vi "Delta Mode Measurements.vi"() -> ()   [LabVIEW 2023]
doc: "Demonstrates the fundamentals of the Queued Message Handler design pattern in LabVIEW. A queued message handler, in its simplest form, is composed of two loops. The Event Handling Loop responds to user interface events by enqueuing \"messages\" on a message queue. These messages are dequeued in the Message Handling Loop. Note that the Message Handling Loop is also capable of sending messages to itself."
uses:
  <instrlib>/Keithley 622x LV 2009/Configure/2182 -A/Low Level/Typedefs/KE2182 -- Voltage Ranges.ctl
  <instrlib>/Keithley 622x LV 2009/Configure/2182 -A/Low Level/Typedefs/KE2182 -- Filter Type.ctl
  <instrlib>/Keithley 622x LV 2009/Configure/2182 -A/Low Level/Typedefs/KE2182 -- Filter Count.ctl
  <instrlib>/Keithley 622x LV 2009/Configure/2182 -A/Low Level/Typedefs/KE2182 -- Filter Window.ctl
  <instrlib>/Keithley 622x LV 2009/Configure/2182 -A/Low Level/Typedefs/KE2182 -- NPLCs.ctl
  <instrlib>/Keithley 622x LV 2009/Configure/Delta PDelta DCon Modes/Typedefs/KE622x -- Delta Mode Params.ctl
  <instrlib>/Keithley 622x LV 2009/Configure/Delta PDelta DCon Modes/Low Level/Typedefs/KE622x -- Delta PDelta Mode High Level.ctl
  <instrlib>/Keithley 622x LV 2009/Configure/Delta PDelta DCon Modes/Low Level/Typedefs/KE622x -- Delta PDelta Mode Low Level.ctl
  <instrlib>/Keithley 622x LV 2009/Configure/Delta PDelta DCon Modes/Low Level/Typedefs/KE622x -- Delta DCon Mode Delay.ctl
  <instrlib>/Keithley 622x LV 2009/Configure/Delta PDelta DCon Modes/Low Level/Typedefs/KE622x -- Delta PDelta Mode Num Cycles Mode.ctl
  <instrlib>/Keithley 622x LV 2009/Configure/Delta PDelta DCon Modes/Low Level/Typedefs/KE622x -- Delta PDelta Mode Num Cycles.ctl
  <instrlib>/Keithley 622x LV 2009/Configure/Units/Typedefs/KE622x -- Voltage Meas Units.ctl
  Program Files/National Instruments/LabVIEW 2023/examples/Design Patterns/Queued Message Handler/support/QMH Fundamentals - Message Cluster.ctl
  <vilib>/Utility/error.llb/Error Cluster From Error Code.vi
  Lakeshore 336/Global temperature.vi
  <vilib>/ErrorRing/Error Ring.xnode
  <instrlib>/Keithley 622x LV 2009/Keithley 622x.lvlib
panel:
  out "Number of points":i32
  out "Array - Numeric":dbl[][](array[numeric]) format="%#_11g"
  out "XY Graph":cluster{dbl[], dbl[]}(graph)
  out "Temperature":dbl format="%.4f"
  in  "Voltage Meas Units":T1
  in  "Stop Delta Mode":bool
  out "Amplitude":dbl
  in  "Exit":bool
  in  "Start Acquisition":bool
  in  "Delta Mode Params In":T2={"High Level (A)"=0.001, "Low Level (A)"=-0.001, "Delay (s)"=0.002, "Num Cycles Mode"=enum."Infinite", "Finite Count"=10, "Abort On\nCompliance?"=FALSE, "Cold Swithing\nMode Enabled?"=FALSE} {"Finite Count" min=2 max=65536; "Low Level (A)" min=-0.105 max=0.0 format="%.3p"; "High Level (A)" min=0.0 max=0.105 format="%.3p"; "Delay (s)" min=0.001 max=9999.999 format="%.3f"}
  in  "2812 -A Params In":T13={"Auto Range?"=FALSE, "Man / Selected\nRange"=enum."10mV", "Enable Digital\nFilter?"=FALSE, "Filter Type"=enum."Moving", "Filter Count"=10, "Filter\nWindow (%)"=0.01, "Enable Analog\nFilter?"=FALSE, "NPLCs"=2} {"Filter\nWindow (%)" min=0.0 max=10.0 step=0.01 format="%.2f"; "Filter Count" min=1 max=100; "NPLCs" min=1 max=10}
  in  "Start Delta Mode":bool
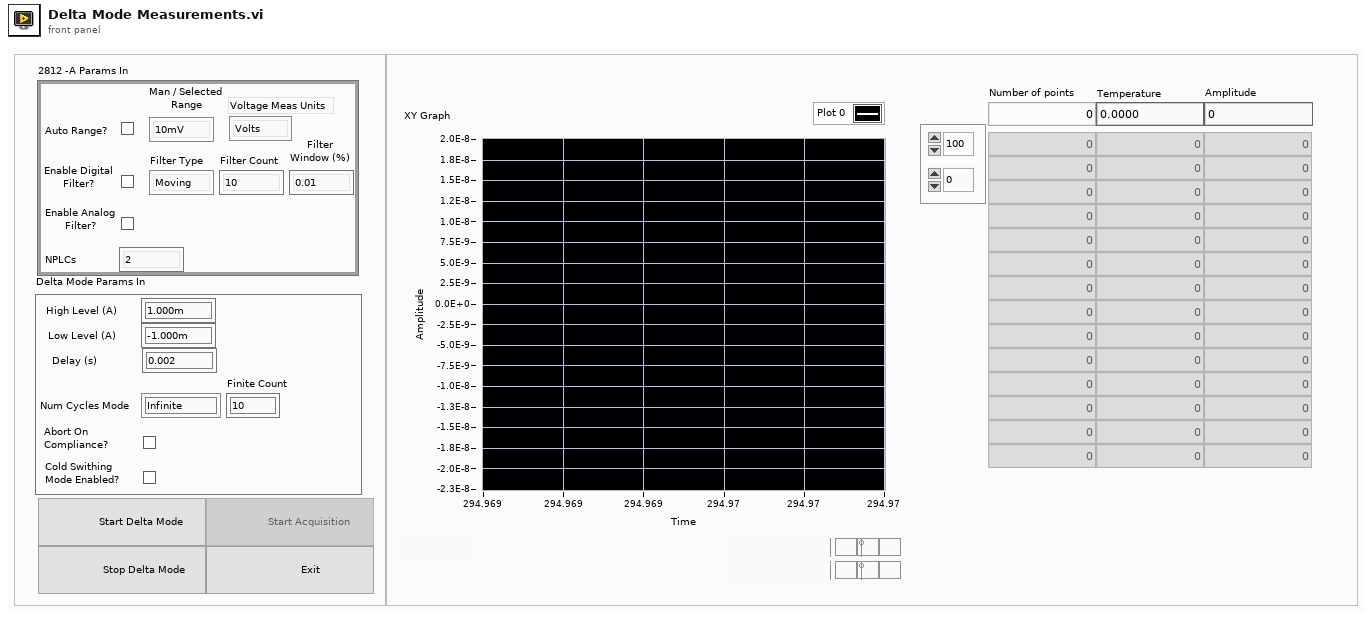
[diagram p1: front panel]
types:
  T1 = typedef "Keithley 622x.lvlib/KE622x -- Voltage Meas Units.ctl" = enum16{"Volts", "Ohms", "Watts", "Siemens"}
  T2 = typedef "Keithley 622x.lvlib/KE622x -- Delta Mode Params.ctl" = cluster{"High Level (A)":T3, "Low Level (A)":T4, "Delay (s)":T5, "Num Cycles Mode":T6, "Finite Count":T7, "Abort On\nCompliance?":bool, "Cold Swithing\nMode Enabled?":bool}
  T3 = typedef "Keithley 622x.lvlib/KE622x -- Delta PDelta Mode High Level.ctl" = dbl
  T4 = typedef "Keithley 622x.lvlib/KE622x -- Delta PDelta Mode Low Level.ctl" = dbl
  T5 = typedef "Keithley 622x.lvlib/KE622x -- Delta DCon Mode Delay.ctl" = dbl
  T6 = typedef "Keithley 622x.lvlib/KE622x -- Delta PDelta Mode Num Cycles Mode.ctl" = enum16{"Finite Count", "Infinite"}
  T7 = typedef "Keithley 622x.lvlib/KE622x -- Delta PDelta Mode Num Cycles.ctl" = u32
  T8 = typedef "Keithley 622x.lvlib/KE2182 -- Voltage Ranges.ctl" = enum16{"10mV", "100mV", "1V", "10V", "100V"}
  T9 = typedef "Keithley 622x.lvlib/KE2182 -- Filter Type.ctl" = enum16{"Moving", "Repeat"}
  T10 = typedef "Keithley 622x.lvlib/KE2182 -- Filter Count.ctl" = u32
  T11 = typedef "Keithley 622x.lvlib/KE2182 -- Filter Window.ctl" = dbl
  T12 = typedef "Keithley 622x.lvlib/KE2182 -- NPLCs.ctl" = u32
  T13 = cluster{"Auto Range?":bool, "Man / Selected\nRange":T8, "Enable Digital\nFilter?":bool, "Filter Type":T9, "Filter Count":T10, "Filter\nWindow (%)":T11, "Enable Analog\nFilter?":bool, "NPLCs":T12}
  T14 = enum8{"Enabled", "Disabled", "Disabled and Grayed Out"}
  T15 = typedef "QMH Fundamentals - Message Cluster.ctl" = cluster{"Message":string, "Message Data":variant}
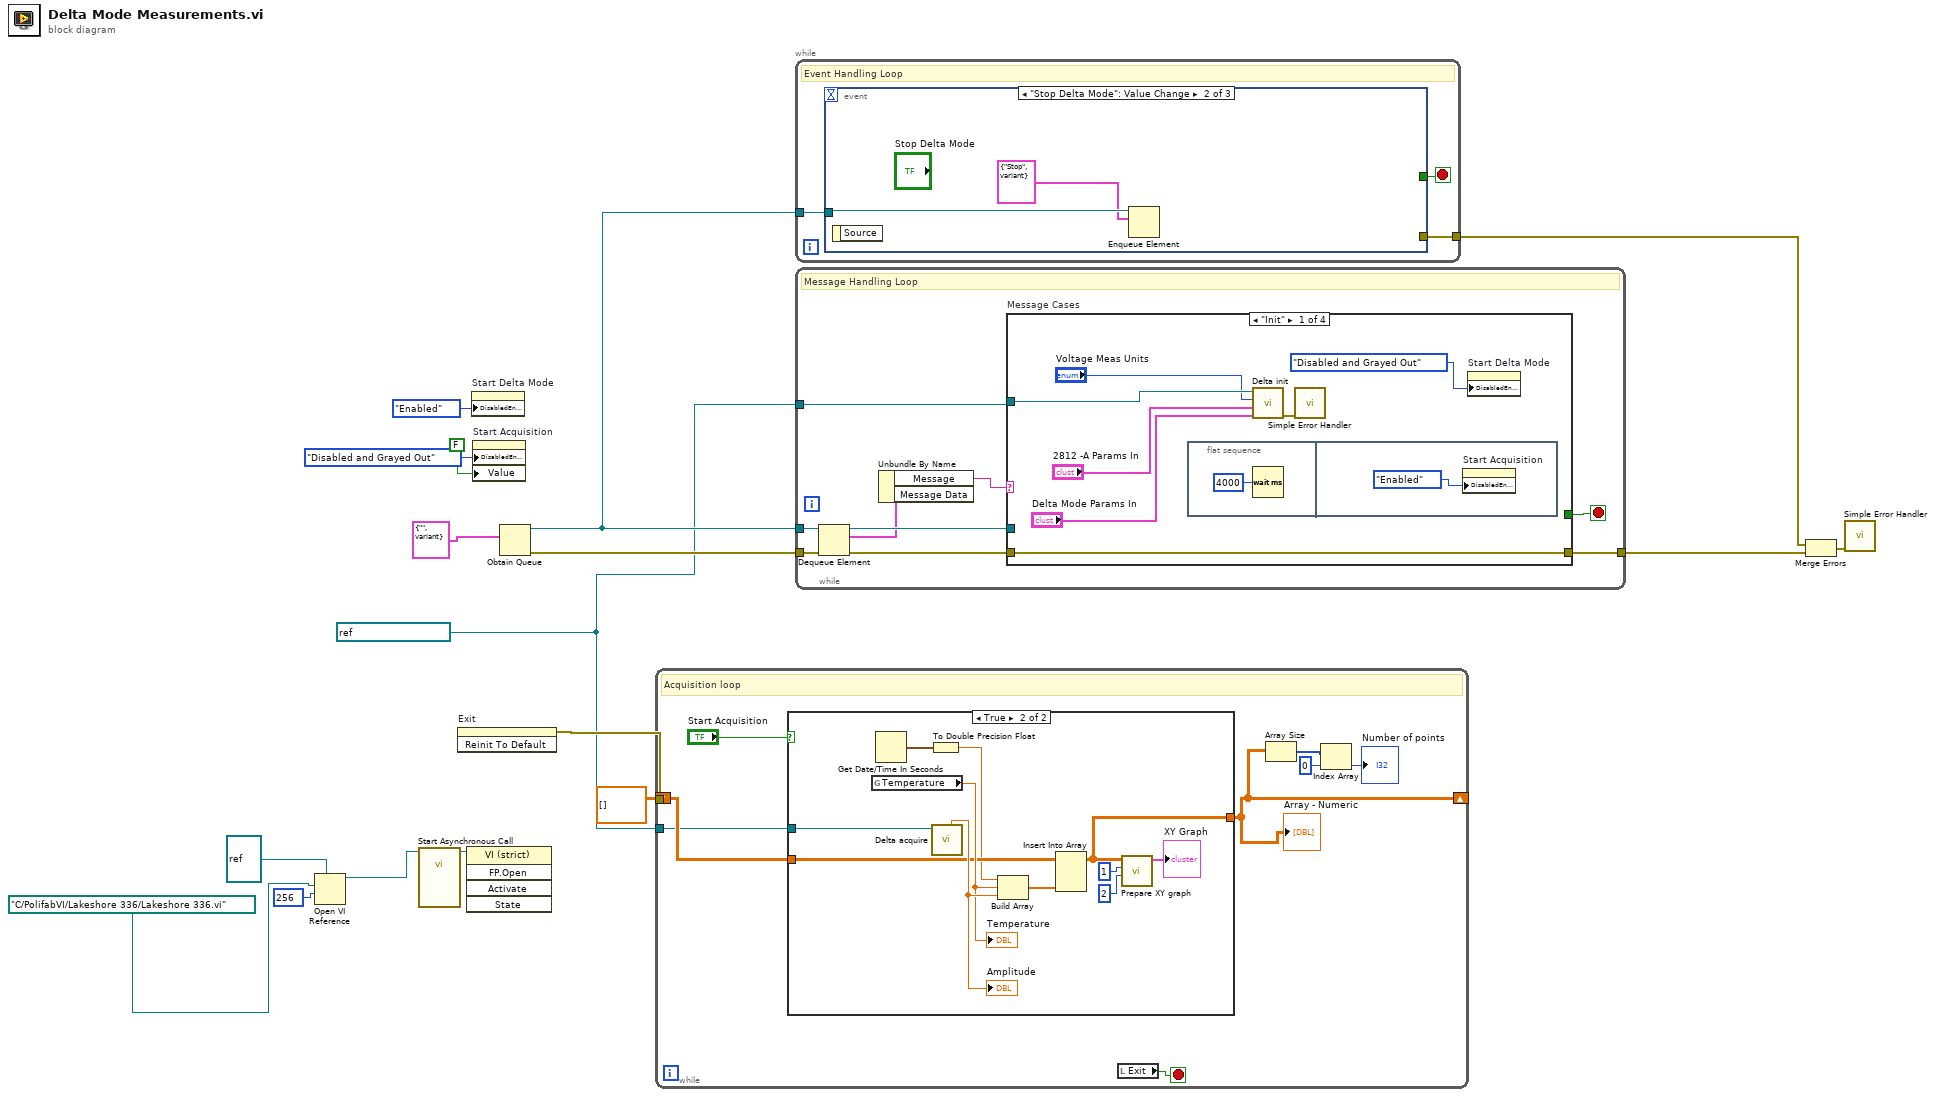
[diagram p0: block diagram]
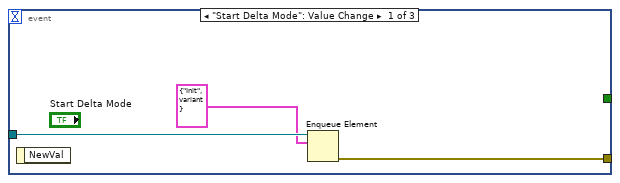
[diagram p3: hidden frame]
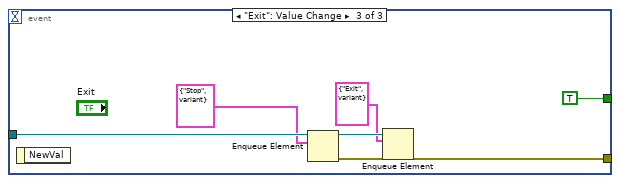
[diagram p4: hidden frame]
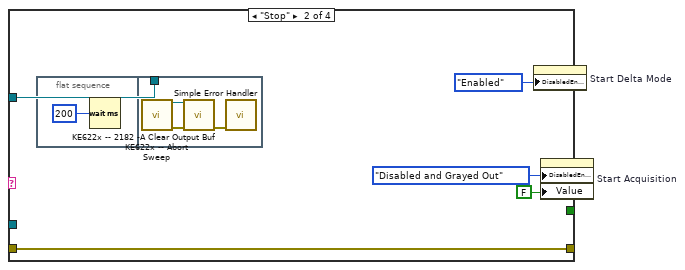
[diagram p5: hidden frame]
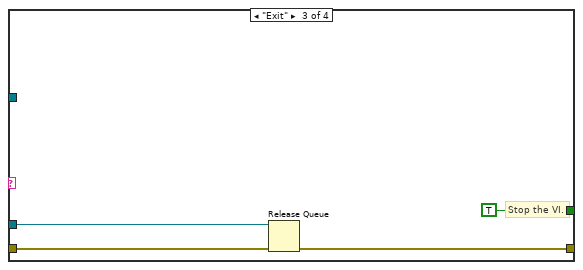
[diagram p6: hidden frame]
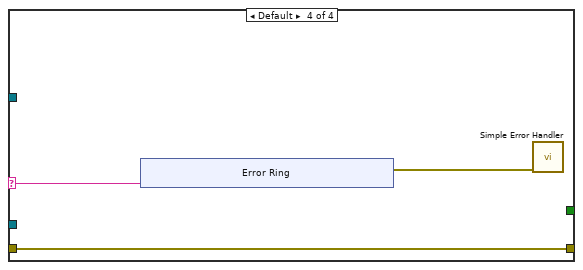
[diagram p7: hidden frame]
diagram:
  w1 = refnum<visa-resource-name> "GPIB0::12::INSTR" ("622x Resource")
  n1 = Open VI Reference(type specifier VI Refnum (for type only)=refnum<vi> refnum, vi path=path "C:/PolifabVI/Lakeshore 336/Lakeshore 336.vi", options=256) -> (vi reference=w4:refnum<vi>)  [unwired: 3 in, 1 out]
  n2 = call-by-ref "Start Asynchronous Call"(reference=w4) -> (reference out=w3:refnum<vi>)  [unwired: 2 in, 2 out]
  n3 = invoke on="Exit" class="Bool (strict)" method="Reinit To Default"() -> (error out=w11:errorcluster)  [unwired: 3 in, 2 out]
  n4 = invoke class="VI (strict)" method="FP.Open"(reference=w3) -> ()  [unwired: 4 in, 5 out]
  n5 = property on="Start Delta Mode" class="Bool"("DisabledEnum"=T14."Enabled" ("Disabled")) -> ()  [unwired: 2 in, 2 out]
  n6 = property on="Start Acquisition" class="Bool (strict)"("DisabledEnum"=T14."Disabled and Grayed Out" ("Disabled"), "Value"=FALSE ("Start Acquisition")) -> ()  [unwired: 2 in, 2 out]
  n7 = Obtain Queue(element data type=T15 {"Message"="", "Message Data"=variant} ("Message Cluster")) -> (queue out=w12:refnum<queue>, error out=w13:errorcluster)  [unwired: 4 in, 1 out]
  n8 = while {
    tunnel: w11 -> [_]
    shift-right: [w21] -> _
    shift-left: dbl[][] [] -> [w23]
    tunnel: w1 -> [w22]
    stop <- w24 stop-if-true
    # "Acquisition loop"
    n9 = case shown="True" "Start Acquisition" {
      tunnel: w23 -> [w26 w34]
      tunnel: [w26 w31] -> w21
      tunnel: w22 -> [_ w27]
      frame False {
      }
      frame True {
        n10 = global read "Global temperature.vi" "Temperature"() -> (w36:dbl)
        "Temperature" <- w36
        n11 = Get Date/Time In Seconds() -> (seconds since 1Jan1904=w28:timestamp)
        n12 = To Double Precision Float(number=w28) -> (double precision float=w29:dbl)
        n13 = call "Delta acquire.vi"("VISA Resource In"=w27) -> ("X Value"=w37:dbl)  [unwired: 7 in, 3 out]
        "Amplitude" <- w37
        n14 = Build Array(w29, w36, w37) -> (w35:dbl[])
        n15 = Insert Into Array(array=w34, new element=w35) -> (w31:dbl[][])  [unwired: 2 in]
        n16 = call "Prepare XY graph.vi"("col2"=2 ("disabled index (col)"), "col1"=1 ("disabled index (col)"), "Array"=w31) -> ("XY"=→"XY Graph":cluster{dbl[], dbl[]})  [unwired: 8 in]
      }
    }
    "Array - Numeric" <- w21
    n17 = local read "Exit"() -> (w24:bool)
    n18 = Array Size(array=w21) -> (size(s)=w20:i32[])
    n19 = Index Array(array=w20, index=0) -> (element=→"Number of points":i32)
  }
  n20 = while {
    tunnel: w12 -> [w40]
    tunnel: [w39] -> w16
    stop <- w38 stop-if-true
    # "Event Handling Loop"
    n21 = event shown="[1] \"Stop Delta Mode\": Value Change" {
      selector: _ -> [_ _ _]
      dyn-events: _ -> [_ _ _]
      timeout: _ -> [_ _ _]
      tunnel: w40 -> [w43 w45 w52]
      tunnel: [w42 _ w46] -> w39
      tunnel: [_ _ TRUE] -> w38
      event "Start Delta Mode": Value Change {
        n22 = event-data() -> ()  [unwired: 1 in, 1 out]
        n23 = Enqueue Element(queue=w43, element=T15 {"Message"="Init", "Message Data"=variant}) -> (error out=w42:errorcluster)  [unwired: 2 in, 2 out]
      }
      event "Stop Delta Mode": Value Change {
        n24 = event-data() -> ()  [unwired: 1 in, 1 out]
        n25 = Enqueue Element(queue=w45, element=T15 {"Message"="Stop", "Message Data"=variant}) -> ()  [unwired: 2 in, 3 out]
      }
      event "Exit": Value Change {
        n26 = event-data() -> ()  [unwired: 1 in, 1 out]
        n27 = Enqueue Element(queue=w52, element=T15 {"Message"="Stop", "Message Data"=variant}) -> (queue out=w48:refnum<queue>, error out=w49:errorcluster)  [unwired: 2 in, 1 out]
        n28 = Enqueue Element(queue=w48, element=T15 {"Message"="Exit", "Message Data"=variant}, error in (no error)=w49) -> (error out=w46:errorcluster)  [unwired: 1 in, 2 out]
      }
    }
  }
  n29 = while {
    tunnel: w12 -> [w58]
    tunnel: w13 -> [w59]
    tunnel: [w60] -> w17
    tunnel: w1 -> [w53]
    stop <- w61 stop-if-true
    # "Message Handling Loop"
    n30 = Dequeue Element(queue=w58, error in (no error)=w59) -> (queue out=w57:refnum<queue>, element=w55:T15, error out=w56:errorcluster)  [unwired: 1 in, 1 out]
    n31 = Unbundle By Name(w55) -> ("Message"=w54:string)  [unwired: 1 out]
    n32 = case "Message Cases" shown="\"Init\"" w54 {
      selector: w54 -> [_ _ _ w87]
      tunnel: w57 -> [_ _ w84 _]
      tunnel: w56 -> [w68 w75 w81 w86]
      tunnel: [w68 w75 w82 w86] -> w60
      tunnel: [_ _ TRUE _] -> w61
      tunnel: w53 -> [w66 w71 _ _]
      frame "Init" {
        n33 = flat-sequence {
          frame #0 {
            n34 = Wait (ms)(milliseconds to wait=u32 4000) -> ()  [unwired: 1 out]
          }
          frame #1 {
            n35 = property on="Start Acquisition" class="Bool (strict)"("DisabledEnum"=T14."Enabled" ("Disabled")) -> ()  [unwired: 2 in, 2 out]
          }
        }
        n36 = call "Delta init.vi"("Delta Mode Params In"="Delta Mode Params In", "2812 -A Params In"="2812 -A Params In", "Voltage Meas Units"="Voltage Meas Units", "VISA Refnum in"=w66) -> ("error out"=w65:errorcluster)  [unwired: 2 in, 1 out]
        n37 = call <vilib>:"Simple Error Handler.vi"("error in (no error)"=w65) -> ()  [unwired: 4 in, 5 out]
        n38 = property on="Start Delta Mode" class="Bool"("DisabledEnum"=T14."Disabled and Grayed Out" ("Disabled")) -> ()  [unwired: 2 in, 2 out]
      }
      frame "Stop" {
        n39 = flat-sequence {
          tunnel: w71 -> [w77]
          frame #0 {
            n40 = Wait (ms)(milliseconds to wait=u32 200) -> ()  [unwired: 1 out]
          }
          frame #1 {
            n41 = call <instrlib>:"KE622x -- Abort Sweep.vi"("Resource In"=w77) -> ("Resource Out (dupl)"=w78:refnum<visa-resource-name>, "error out"=w79:errorcluster)  [unwired: 13 in]
            n42 = call <instrlib>:"KE622x -- 2182 -A Clear Output Buf.vi"("622x Resource In"=w78, "error in (no error)"=w79) -> ("error out"=w80:errorcluster)  [unwired: 11 in, 2 out]
            n43 = call <vilib>:"Simple Error Handler.vi"("error in (no error)"=w80) -> ()  [unwired: 4 in, 5 out]
          }
        }
        n44 = property on="Start Delta Mode" class="Bool"("DisabledEnum"=T14."Enabled" ("Disabled")) -> ()  [unwired: 2 in, 2 out]
        n45 = property on="Start Acquisition" class="Bool (strict)"("DisabledEnum"=T14."Disabled and Grayed Out" ("Disabled"), "Value"=FALSE ("Start Acquisition")) -> ()  [unwired: 2 in, 2 out]
      }
      frame "Exit" {
        # "Stop the VI."
        # "Exit - Exit the application. Since this message was sent as a priority message (i.e., it was placed at the front of the queue), any cleanup code should run here, since the loop is about to stop. Any other messages in the queue will not be handled."
        n46 = Release Queue(queue=w84, error in (no error)=w81) -> (error out=w82:errorcluster)  [unwired: 1 in, 2 out]
      }
      frame Default {
        # "The Default case only runs if there is a message that isn't defined in any of the other cases. Generate an error if this occurs."
        n47 = xnode "Error Ring"("parameter 0"=w87) -> ("error out"=w85:errorcluster)
        n48 = call <vilib>:"Simple Error Handler.vi"("error in (no error)"=w85) -> ()  [unwired: 4 in, 5 out]
      }
    }
  }
  n49 = Merge Errors(w16, w17) -> (w15:errorcluster)
  n50 = call <vilib>:"Simple Error Handler.vi"("error in (no error)"=w15) -> ()  [unwired: 4 in, 5 out]
